vi "Win32 Window Handle Wrapper.vi"(8 "error in (no error)":errorcluster, 10 "WindowWrapper DLL Directory":path, 11 "Win32 Window Handle":i32) -> (0 "error out":errorcluster, 3 "System.Windows.Forms.IWin32Window":refnum<k24>)   [LabVIEW 2013, in "Win32 Util.lvlib"]
doc: "This VI Creates a IWin32Window Typed reference a the Win32 Windows Handle."
uses:
  Win32 Util.lvlib
  System.Windows.Forms
  C:/dev/Kraft/DX Data Logger 1/Source/HMI/Re-use Libraries/Win32 Util/WindowWrapper.dll
  WindowWrapper.dll
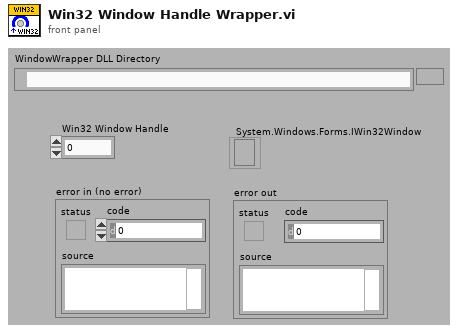
[diagram p1: front panel]
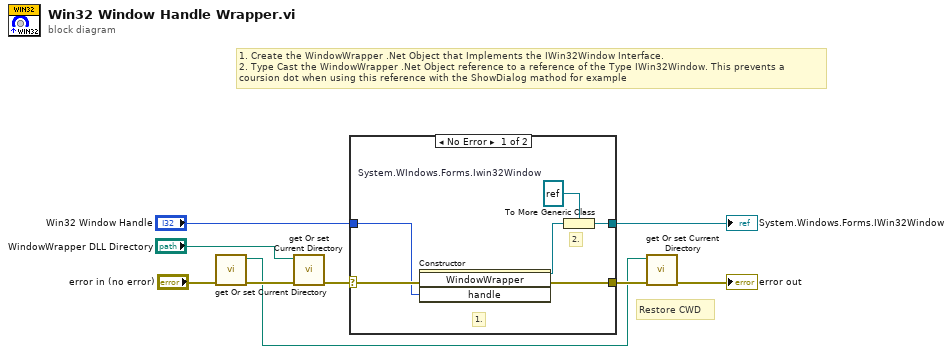
[diagram p0: block diagram]
diagram:
  # "Restore CWD"
  # "1. Create the WindowWrapper .Net Object that Implements the IWin32Window Interface.\n2. Type Cast the WindowWrapper .Net Object reference to a reference of the Type IWin32Window. This prevents a \ncoursion dot when using this reference with the ShowDialog mathod for example"
  n1 = call "get Or set Current Directory.vi"("error in (no error)"="error in (no error)") -> ("error out"=w4:errorcluster, "Get Directory"=w3:path)  [unwired: 9 in]
  n2 = call "get Or set Current Directory.vi"("error in (no error)"=w4, "Set Directory"="WindowWrapper DLL Directory") -> ("error out"=w7:errorcluster)  [unwired: 8 in, 1 out]
  n3 = case shown="No Error" w7 {
    selector: w7 -> [w11 w16]
    tunnel: "Win32 Window Handle" -> [w10 _]
    tunnel: [w12 w16] -> w6
    tunnel: [w13 _] -> w8
    frame No Error {
      w15 = refnum<k24> refnum  # System.WIndows.Forms.Iwin32Window
      # "2."
      # "1."
      n4 = constructor class="WindowWrapper"(error in=w11, "handle"=w10) -> (reference out=w14:refnum<k24>, error out=w12:errorcluster)  [unwired: 2 in, 2 out]
      n5 = To More Generic Class(target class=w15, reference=w14) -> (generic class reference=w13:refnum<k24>)
    }
    frame Error {
    }
  }
  "System.Windows.Forms.IWin32Window" <- w8
  n6 = call "get Or set Current Directory.vi"("error in (no error)"=w6, "Set Directory"=w3) -> ("error out"=→"error out":errorcluster)  [unwired: 8 in, 1 out]
